vi "CheesyDrive.vi"(6 "Quickturn":bool, 7 "SlowMode":u32, 10 "Wheel":dbl(slide)=-0.023622047244094488 scale=-1.0..1.0, 11 "Throttle":dbl(slide)=0.007874015748031496 scale=-1.0..1.0) -> (2 "Right PWM":dbl, 3 "Left PWM":dbl)   [LabVIEW 2020]
doc: "Implements CheesyDrive. CheesyDrive means that the turn joystick controls the radius of turning instead of the rate of turning. Also implements QuickStop and QuickTurn."
panel:
  in  "ArrayOfSlownesss":T1(array[cluster])=[{"MaxSpeedSlow"=1.0, "SlowRate"=5.0, "MaxTurnSlow"=1.0, "MaxTurnRateSlow"=10.0}, {"MaxSpeedSlow"=0.6, "SlowRate"=4.0, "MaxTurnSlow"=0.8, "MaxTurnRateSlow"=10.0}, {"MaxSpeedSlow"=0.4, "SlowRate"=3.0, "MaxTurnSlow"=0.75, "MaxTurnRateSlow"=10.0}]
  in  "PointsTurn":cluster{"X":dbl, "Y":dbl}[](array[cluster])=[{"X"=0.0, "Y"=0.0}, {"X"=0.04, "Y"=0.0}, {"X"=0.041, "Y"=0.01}, {"X"=1.0, "Y"=1.0}]
  in  "PointsQuickTurn":cluster{"X":dbl, "Y":dbl}[](array[cluster])=[{"X"=0.0, "Y"=0.0}, {"X"=0.04, "Y"=0.0}, {"X"=0.8, "Y"=0.7}, {"X"=1.0, "Y"=1.0}]
  in  "PointsThrottle":cluster{"X":dbl, "Y":dbl}[](array[cluster])=[{"X"=0.0, "Y"=0.0}, {"X"=0.04, "Y"=0.0}, {"X"=0.0251, "Y"=0.15}, {"X"=1.0, "Y"=1.0}]
  in  "QSMult":dbl=0.15
  in  "WheelNonLinearity":dbl=0.65
  in  "negInertiaScalar":dbl=3.0
  in  "alpha":dbl=0.1
  out "Waveform Chart":dbl(graph)
  in  "Sensitivty":dbl=1.0
  # "Enable to enable"
  # "normal"
  # "(for quickstop decay)"
  # "Switch"
  # "Scale"
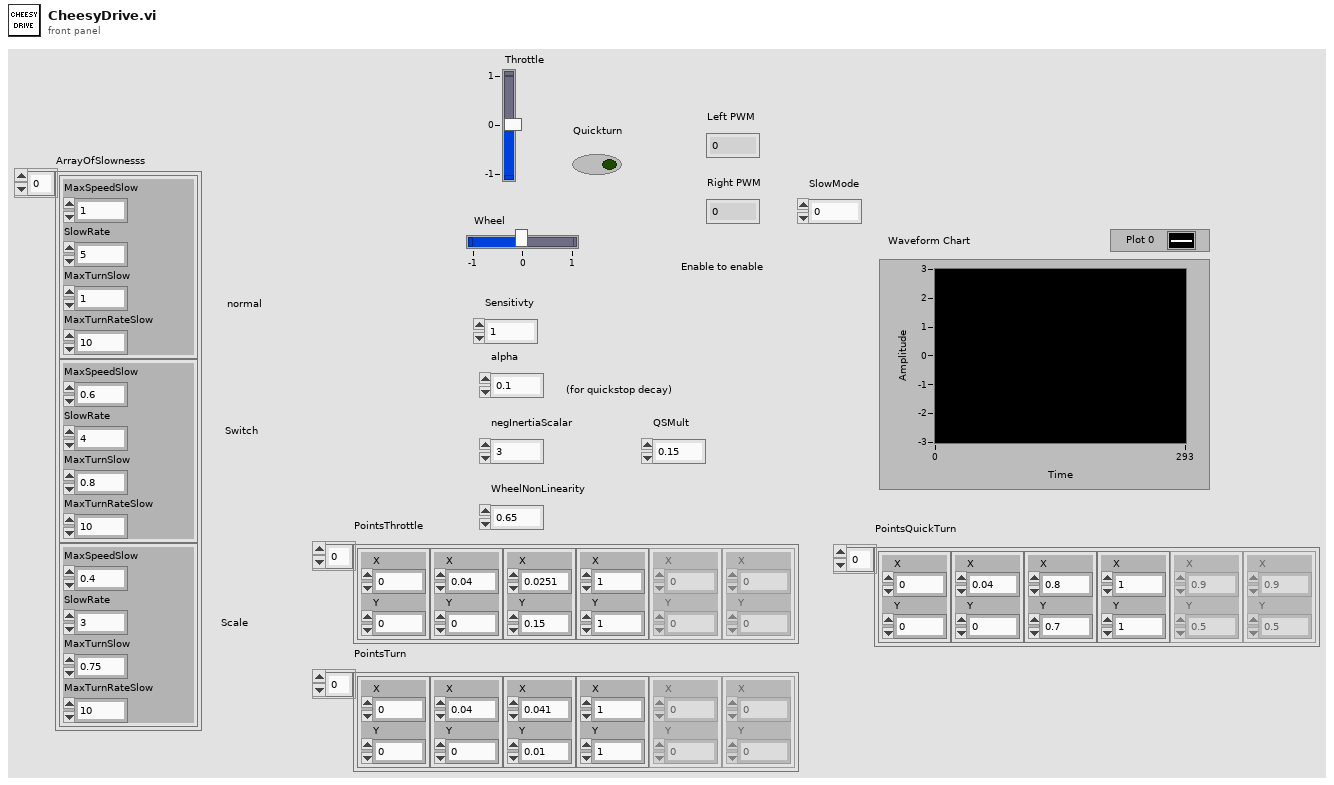
[diagram p1: front panel]
types:
  T1 = cluster{"MaxSpeedSlow":dbl, "SlowRate":dbl, "MaxTurnSlow":dbl, "MaxTurnRateSlow":dbl}[]
  T2 = cluster{"MaxSpeedSlow":dbl, "SlowRate":dbl, "MaxTurnSlow":dbl, "MaxTurnRateSlow":dbl}
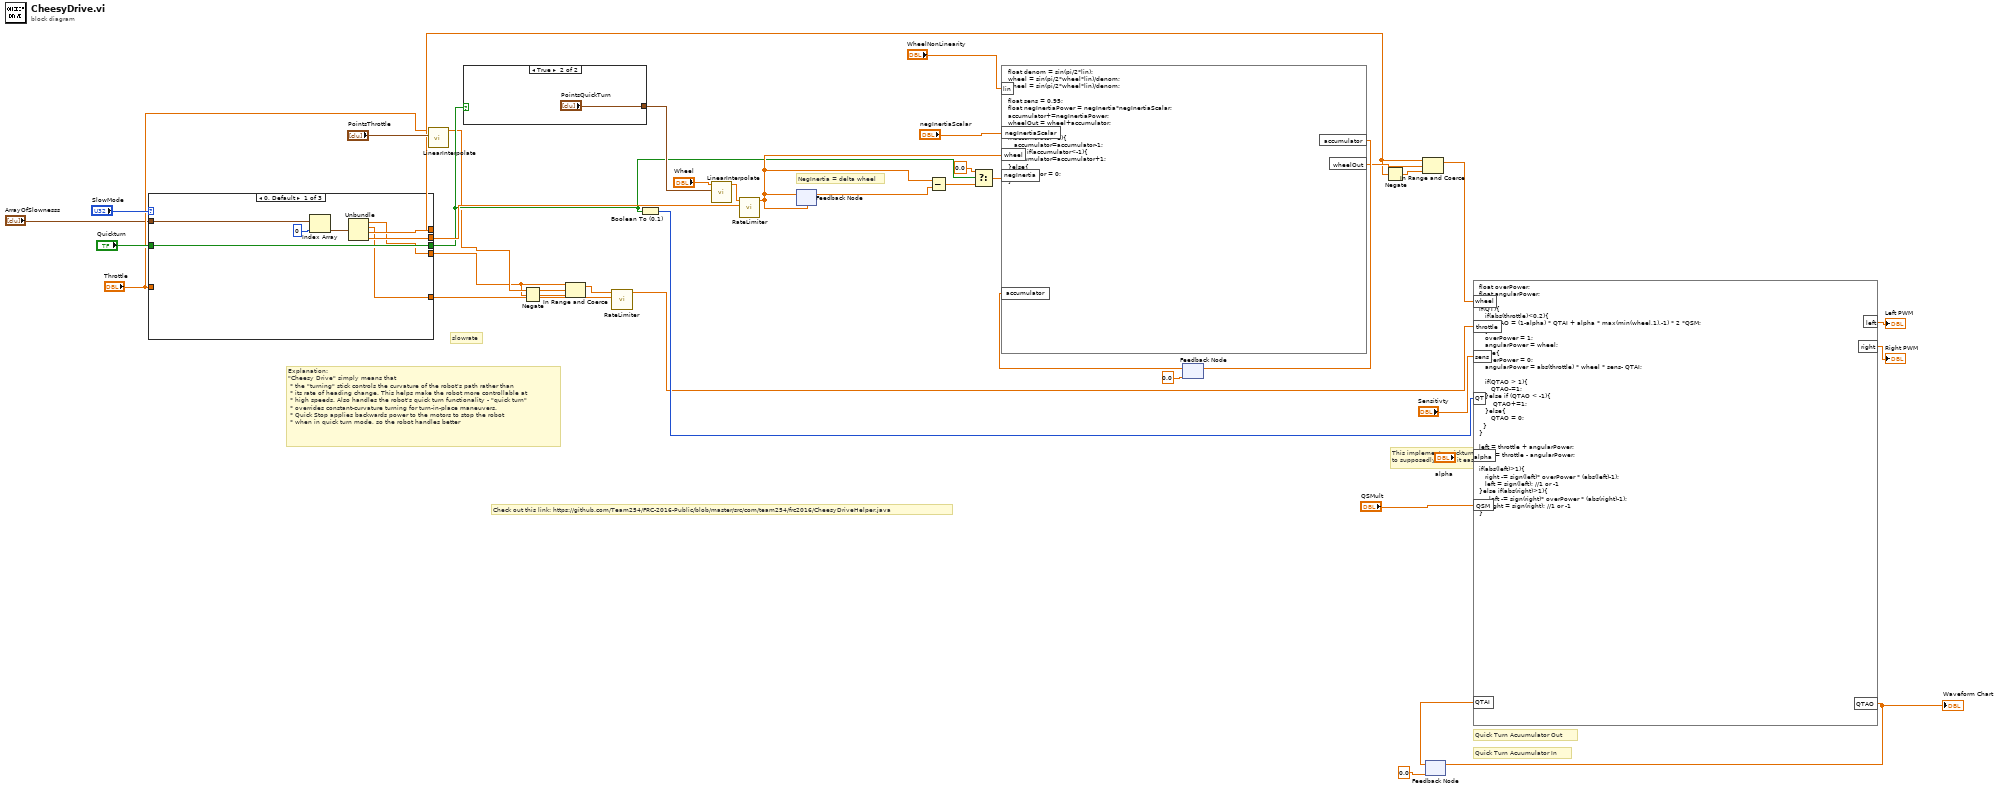
[diagram p0: block diagram]
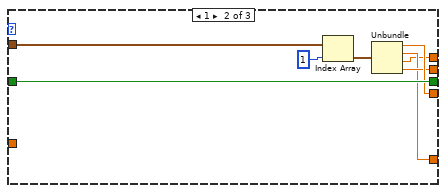
[diagram p2: hidden frame]
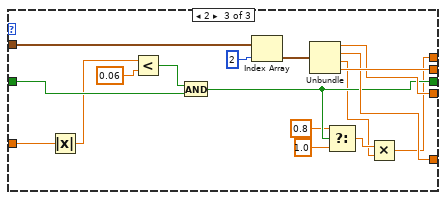
[diagram p3: hidden frame]
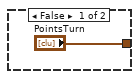
[diagram p4: hidden frame]
diagram:
  # "slowrate"
  # "This implements quickturn and also modifies wheel with a sine function\nto supposedly make it easier to drive"
  # "NegInertia = delta wheel"
  # "Explanation:\n\"Cheesy Drive\" simply means that\n * the \"turning\" stick controls the curvature of the robot's path rather than\n * its rate of heading change. This helps make the robot more controllable at\n * high speeds. Also handles the robot's quick turn functionality - \"quick turn\"\n * overrides constant-curvature turning for turn-in-place maneuvers.\n * Quick Stop applies backwards power to the motors to stop the robot\n * when in quick turn mode, so the robot handles better"
  # "Quick Turn Acuumulator Out"
  # "Quick Turn Acuumulator In"
  # "Check out this link: https://github.com/Team254/FRC-2016-Public/blob/master/src/com/team254/frc2016/CheesyDriveHelper.java"
  n1 = case shown="0, Default" "SlowMode" {
    tunnel: [w40 w49 w63] -> w17
    tunnel: [w41 w51 w65] -> w1
    tunnel: [w42 w48 w56] -> w15
    tunnel: [w43 w50 w66] -> w13
    tunnel: "Quickturn" -> [w47 w55 w72]
    tunnel: [w47 w55 w60] -> w6
    tunnel: "Throttle" -> [_ _ w64]
    tunnel: "ArrayOfSlownesss" -> [w44 w52 w69]
    frame 0, Default {
      n2 = Index Array(array=w44, index=0) -> (element=w45:T2)
      n3 = Unbundle(w45) -> ("MaxSpeedSlow"=w41:dbl, "SlowRate"=w40:dbl, "MaxTurnSlow"=w42:dbl, "MaxTurnRateSlow"=w43:dbl)
    }
    frame 1 {
      n4 = Index Array(array=w52, index=1) -> (element=w53:T2)
      n5 = Unbundle(w53) -> ("MaxSpeedSlow"=w51:dbl, "SlowRate"=w49:dbl, "MaxTurnSlow"=w48:dbl, "MaxTurnRateSlow"=w50:dbl)
    }
    frame 2 {
      n6 = Absolute Value(x=w64) -> (abs(x)=w62:dbl)
      n7 = Less?(x=w62, y=0.06) -> (x < y?=w71:bool)
      n8 = And(x=w71, y=w72) -> (x .and. y?=w60:bool)
      n9 = Index Array(array=w69, index=2) -> (element=w67:T2)
      n10 = Unbundle(w67) -> ("MaxSpeedSlow"=w65:dbl, "SlowRate"=w63:dbl, "MaxTurnSlow"=w57:dbl, "MaxTurnRateSlow"=w66:dbl)
      n11 = Select(t=0.8, s=w60, f=1.0) -> (s? t:f=w58:dbl)
      n12 = Multiply(x=w58, y=w57) -> (x*y=w56:dbl)
    }
  }
  n13 = call "LinearInterpolate.vi"("Points"="PointsThrottle", "Value"="Throttle") -> ("Output"=w3:dbl)  [unwired: 9 in]
  n14 = case shown="True" w6 {
    tunnel: ["PointsTurn" "PointsQuickTurn"] -> w19
    frame False {
    }
    frame True {
    }
  }
  n15 = Negate(x=w1) -> (-x=w2:dbl)
  n16 = In Range and Coerce(upper limit=w1, x=w3, lower limit=w2) -> (coerced(x)=w4:dbl)  [unwired: 1 out]
  n17 = call "RateLimiter.vi"("Max dx/dt"=w17, "Input"=w4) -> ("Output"=w33:dbl)  [unwired: 9 in]
  n18 = Boolean To (0,1)(Boolean=w6) -> (0, 1=w37:i16)
  n19 = call "LinearInterpolate.vi"("Points"=w19, "Value"="Wheel") -> ("Output"=w14:dbl)  [unwired: 9 in]
  n20 = call "RateLimiter.vi"("Max dx/dt"=w13, "Input"=w14) -> ("Output"=w21:dbl)  [unwired: 9 in]
  n21 = feedback #1(w21) -> (w30:dbl)
  n22 = feedback-in #1(w21) -> ()
  n23 = Subtract(x=w21, y=w30) -> (x-y=w11:dbl)
  n24 = Select(t=0.0, s=w6, f=w11) -> (s? t:f=w12:dbl)
  n25 = feedback #2(0.0 ("Wheel")) -> (w29:dbl)
  n26 = formula code="float denom = sin(pi/2*lin);\nwheel = sin(pi/2*wheel*lin)/denom;\nwheel = sin(pi/2*wheel*lin)/denom;\n\nfloat sens = 0.95;\nfloat negInertiaPower = negInertia*negInertiaScalar;\naccumulator+=negInertiaPower;\nwheelOut = wheel+accumulator;\n\nif(accumulator>1){\n   accumulator=accumulator-1;\n}else if(accumulator<-1){\n   accumulator=accumulator+1;\n}else{\naccumulator = 0;\n}"("wheel"=w21, "negInertia"=w12, "accumulator"=w29, "negInertiaScalar"="negInertiaScalar", "lin"="WheelNonLinearity") -> ("accumulator"=w27:dbl, "wheelOut"=w23:dbl)
  n27 = feedback-in #2(w27) -> ()
  n28 = Negate(x=w15) -> (-x=w16:dbl)
  n29 = In Range and Coerce(upper limit=w15, x=w23, lower limit=w16) -> (coerced(x)=w24:dbl)  [unwired: 1 out]
  n30 = feedback #3(0.0 ("QTAccumulatorO")) -> (w35:dbl)
  n31 = formula code="float overPower;\nfloat angularPower;\n\nif(QT){\n   if(abs(throttle)<0.2){\n      QTAO = (1-alpha) * QTAI + alpha * max(min(wheel,1),-1) * 2 *QSM;\n   }\n   overPower = 1;\n   angularPower = wheel;\n}else{\n   overPower = 0;\n   angularPower = abs(throttle) * wheel * sens- QTAI;\n\n   if(QTAO > 1){\n      QTAO-=1;\n   }else if (QTAO < -1){\n       QTAO+=1;\n   }else{\n      QTAO = 0;\n  }\n}\n\nleft = throttle + angularPower;\nright = throttle - angularPower;\n\nif(abs(left)>1){\n   right -= sign(left)* overPower * (abs(left)-1);\n   left = sign(left); //1 or -1\n}else if(abs(right)>1){\n     left -= sign(right)* overPower * (abs(right)-1);\n     right = sign(right); //1 or -1 \n}"("wheel"=w24, "throttle"=w33, "sens"="Sensitivty", "QT"=w37, "alpha"="alpha", "QTAI"=w35, "QSM"="QSMult") -> ("left"=→"Left PWM":dbl, "right"=→"Right PWM":dbl, "QTAO"=w38:dbl)
  "Waveform Chart" <- w38
  n32 = feedback-in #3(w38) -> ()
